vi "Pre Launch Init.vi"(11 "Rack Controller in":refnum<class "Rack Controller.lvclass">) -> (0 "error out":errorcluster, 3 "Rack Controller out":refnum<class "Rack Controller.lvclass">)   [LabVIEW 2019, in "Rack Controller.lvclass"]
doc: "(<B>Filename</B>: Actor Framework.lvlib:Actor.lvclass:Pre Launch Init.vi)\n\nDefines behavior that occurs after the Launch Nested Actor method is invoked but before the actor's Actor Core method begins running.\n\nBy default, this method does nothing. A descendant class may override it to define behavior."
uses:
  Rack Controller.lvclass
  <vilib>/ActorFramework/Message Enqueuer/Message Enqueuer.lvclass
  <vilib>/vision/Image Controls.llb/IMAQ Image.ctl
  <vilib>/ActorFramework/Actor/Actor.lvclass
  Common/Controls/Acknowledgement.ctl
  Common/Controls/Camera Optics Diagnostics.ctl
  Common/Controls/Camera Optics Diagnostics Result.ctl
  Common/Controls/Camera Info.ctl
  Inspection Statemachine/Controls/Result Cluster_SM.ctl
  Inspection Statemachine/Inspection Statemachine.lvclass
  Controls/Result Cluster_RC.ctl
  Common/Controls/AllPartInfo.ctl
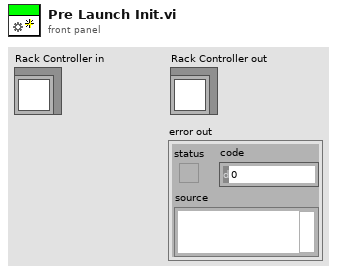
[diagram p1: front panel]
types:
  T1 = typedef "IMAQ Image.ctl" = refnum<image>
  T2 = typedef "AllPartInfo.ctl" = cluster{"PartName":string, "NumberOfRacks":u8, "MeasurementIDsArray":u16[], "MeasurementNamesArray":string[], "SpecValuesArray":cluster{"LCL":dbl, "UCL":dbl, "LSL":dbl, "USL":dbl, "NominalValue":dbl}[]}[]
  T3 = cluster{"PartName":string, "MeasurementIDsArray":u16[], "MeasurementNamesArray":string[], "SpecValuesArray":cluster{"LCL":dbl, "UCL":dbl, "LSL":dbl, "USL":dbl, "NominalValue":dbl}[]}
  T4 = cluster{"Unload Position Counts":cluster{"Fail":u32, "ReelEnd":u32, "ProductionEnd":u32}, "Number of Cameras":u8}
  T5 = cluster{"Result Cluster":cluster{"Rack ID":u8, "Measurement Values Array ":dbl[], "Images Array":T1[], "Result PF":bool, "Production Count Details":cluster{"Total Fail":u64, "Total Pass":u64, "Total Count":u64}, "Reel Count Details":cluster{"Reel Fail":u64, "Reel Pass":u64, "Reel Count":u64}, "Control PF Array":bool[], "Specification PF Array":bool[], "Specification Fail?":bool, "Reel Number":u64, "Status":string}, "Pause on Fail?":bool, "Total Count Finish?":bool, "Reel Count Finish?":bool}
  T6 = typedef "Inspection Statemachine.lvclass/Result Cluster_SM.ctl" = cluster{"RackID":u8, "MeasurementValuesArray ":dbl[], "ImagesArray":T1[], "ResultPF":bool, "ProductionCountDetails":cluster{"TotalFail":u64, "TotalPass":u64, "TotalCount":u64}, "ReelCountDetails":cluster{"ReelFail":u64, "ReelPass":u64, "ReelCount":u64}, "ControlPFArray":bool[], "SpecificationPFArray":bool[], "SpecificationFail":bool, "ReelNumber":u64, "Status":string}
  T7 = cluster{"Part Name":string, "Total Count":u64, "Reel Count":u64}
  T8 = typedef "Camera Info.ctl" = cluster{"Camera Names":string[], "Number of Active Cameras":u8}
  T9 = typedef "Camera Optics Diagnostics Result.ctl" = cluster{"LightCameraName":string, "DiagnosedImage":T1, "DustPercentage":dbl, "Result":bool}
  T10 = typedef "Camera Optics Diagnostics.ctl" = cluster{"Light Camera Name":string, " State":string}
  T11 = typedef "Rack Controller.lvclass/Result Cluster_RC.ctl" = cluster{"Measurement Values Array ":dbl[], "Images Array":T1[], "Result PF":bool, "Production Count Details":cluster{"Total Fail":u64, "Total Pass":u64, "Total Count":u64}, "Reel Count Details":cluster{"Reel Fail":u64, "Reel Pass":u64, "Reel Count":u64}, "Control PF Array":bool[], "Specification PF Array":bool[], "Specification Fail?":bool}
  T12 = typedef "Acknowledgement.ctl" = cluster{"Enqueuer":refnum<class "Message Enqueuer.lvclass">, "VIReference":refnum<vi>, "VIName":string}
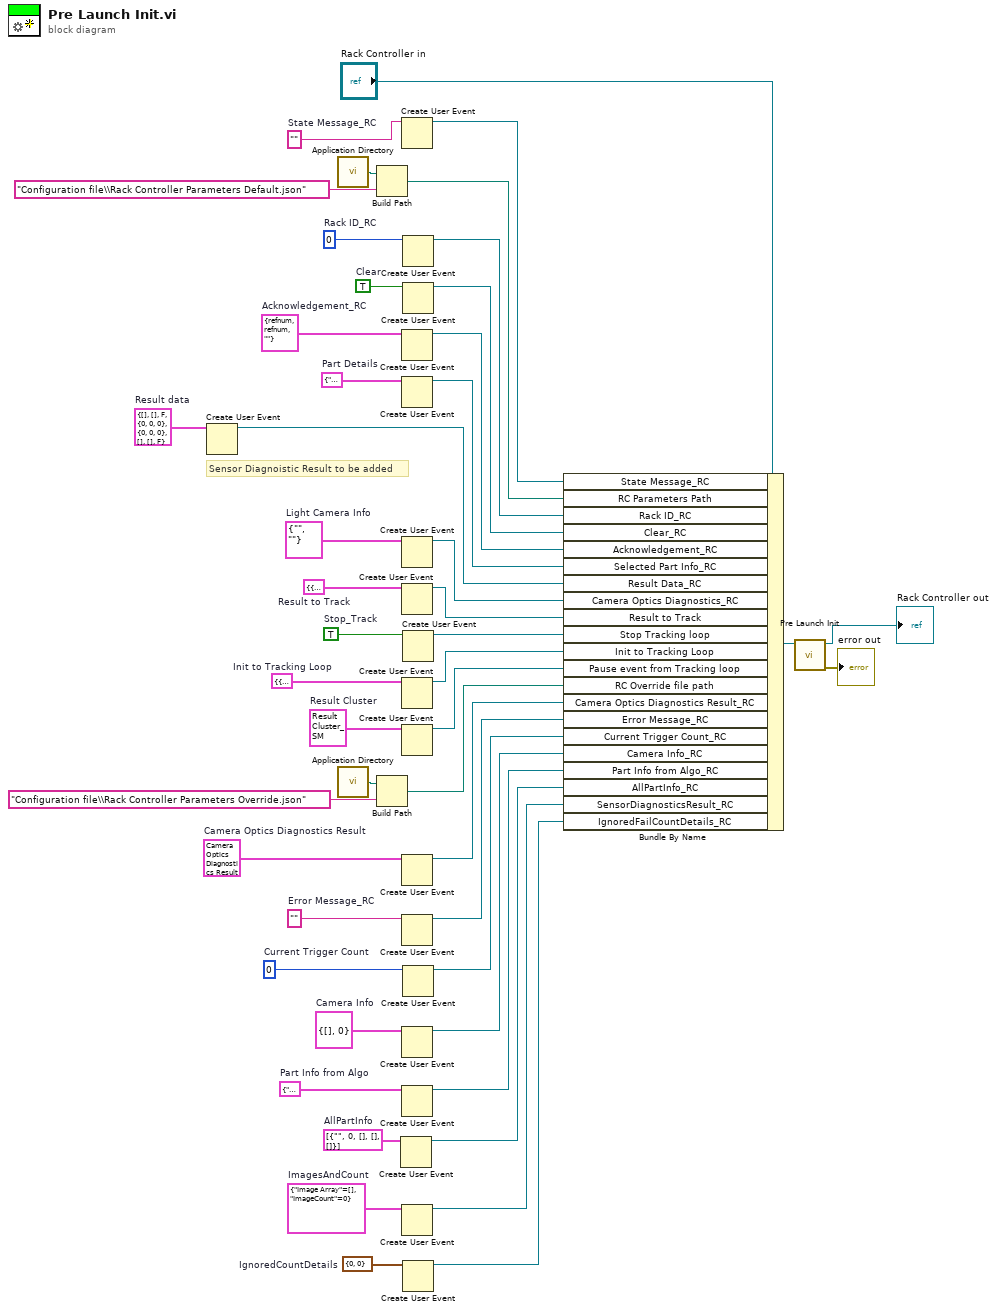
[diagram p0: block diagram]
diagram:
  w2 = cluster{"ReelCount":u64, "TotalCount":u64} {"ReelCount"=0, "TotalCount"=0}  # IgnoredCountDetails
  w4 = cluster{"Image Array":T1[], "ImageCount":u64} {"Image Array"=[], "ImageCount"=0}  # ImagesAndCount
  w6 = T2 [{"PartName"="", "NumberOfRacks"=0, "MeasurementIDsArray"=[], "MeasurementNamesArray"=[], "SpecValuesArray"=[]}]  # AllPartInfo
  w8 = T3 {"PartName"="", "MeasurementIDsArray"=[], "MeasurementNamesArray"=[], "SpecValuesArray"=[]}  # Part Info from Algo
  w13 = T4 {"Unload Position Counts"={"Fail"=0, "ReelEnd"=0, "ProductionEnd"=0}, "Number of Cameras"=0}  # Init to Tracking Loop
  w15 = T5 {"Result Cluster"={"Rack ID"=0, "Measurement Values Array "=[], "Images Array"=[], "Result PF"=FALSE, "Production Count Details"={"Total Fail"=0, "Total Pass"=0, "Total Count"=0}, "Reel Count Details"={"Reel Fail"=0, "Reel Pass"=0, "Reel Count"=0}, "Control PF Array"=[], "Specification PF Array"=[], "Specification Fail?"=FALSE, "Reel Number"=0, "Status"=""}, "Pause on Fail?"=TRUE, "Total Count Finish?"=FALSE, "Reel Count Finish?"=FALSE}  # Result to Track
  w11 = T6 {"RackID"=0, "MeasurementValuesArray "=[], "ImagesArray"=[], "ResultPF"=FALSE, "ProductionCountDetails"={"TotalFail"=0, "TotalPass"=0, "TotalCount"=0}, "ReelCountDetails"={"ReelFail"=0, "ReelPass"=0, "ReelCount"=0}, "ControlPFArray"=[], "SpecificationPFArray"=[], "SpecificationFail"=FALSE, "ReelNumber"=0, "Status"=""}  # Result Cluster
  w18 = T7 {"Part Name"="", "Total Count"=0, "Reel Count"=0}  # Part Details
  w21 = T8 {"Camera Names"=[], "Number of Active Cameras"=0}  # Camera Info
  w25 = T9 {"LightCameraName"="", "DiagnosedImage"=refnum, "DustPercentage"=0.0, "Result"=TRUE}  # Camera Optics Diagnostics Result
  w29 = u64 0  # Current Trigger Count
  w31 = ""  # Error Message_RC
  w36 = TRUE  # Stop_Track
  w37 = T10 {"Light Camera Name"="", " State"=""}  # Light Camera Info
  w10 = T11 {"Measurement Values Array "=[], "Images Array"=[], "Result PF"=FALSE, "Production Count Details"={"Total Fail"=0, "Total Pass"=0, "Total Count"=0}, "Reel Count Details"={"Reel Fail"=0, "Reel Pass"=0, "Reel Count"=0}, "Control PF Array"=[], "Specification PF Array"=[], "Specification Fail?"=FALSE}  # Result data
  w41 = T12 {"Enqueuer"=refnum, "VIReference"=refnum, "VIName"=""}  # Acknowledgement_RC
  w42 = TRUE  # Clear
  w43 = 0  # Rack ID_RC
  w44 = ""  # State Message_RC
  # "Sensor Diagnoistic Result to be added"
  n1 = Create User Event(user event datatype=w10) -> (user event=w28:refnum<user-event>)  [unwired: 1 in, 1 out]
  n2 = call <vilib>:"Application Directory.vi"() -> ("Application Directory"=w40:path)
  n3 = call <vilib>:"Application Directory.vi"() -> ("Application Directory"=w34:path)
  n4 = Build Path(base path=w40, name or relative path="Configuration file\\Rack Controller Parameters Default.json") -> (appended path=w38:path)
  n5 = Build Path(base path=w34, name or relative path="Configuration file\\Rack Controller Parameters Override.json") -> (appended path=w32:path)
  n6 = Create User Event(user event datatype=w6) -> (user event=w5:refnum<user-event>)  [unwired: 1 in, 1 out]
  n7 = Create User Event(user event datatype=w44) -> (user event=w19:refnum<user-event>)  [unwired: 1 in, 1 out]
  n8 = Create User Event(user event datatype=w41) -> (user event=w27:refnum<user-event>)  [unwired: 1 in, 1 out]
  n9 = Create User Event(user event datatype=w18) -> (user event=w17:refnum<user-event>)  [unwired: 1 in, 1 out]
  n10 = Create User Event(user event datatype=w37) -> (user event=w26:refnum<user-event>)  [unwired: 1 in, 1 out]
  n11 = Create User Event(user event datatype=w15) -> (user event=w14:refnum<user-event>)  [unwired: 1 in, 1 out]
  n12 = Create User Event(user event datatype=w13) -> (user event=w12:refnum<user-event>)  [unwired: 1 in, 1 out]
  n13 = Create User Event(user event datatype=w11) -> (user event=w16:refnum<user-event>)  [unwired: 1 in, 1 out]
  n14 = Create User Event(user event datatype=w25) -> (user event=w24:refnum<user-event>)  [unwired: 1 in, 1 out]
  n15 = Create User Event(user event datatype=w31) -> (user event=w30:refnum<user-event>)  [unwired: 1 in, 1 out]
  n16 = Create User Event(user event datatype=w21) -> (user event=w20:refnum<user-event>)  [unwired: 1 in, 1 out]
  n17 = Create User Event(user event datatype=w8) -> (user event=w7:refnum<user-event>)  [unwired: 1 in, 1 out]
  n18 = Create User Event(user event datatype=w4) -> (user event=w3:refnum<user-event>)  [unwired: 1 in, 1 out]
  n19 = Create User Event(user event datatype=w43) -> (user event=w23:refnum<user-event>)  [unwired: 1 in, 1 out]
  n20 = Create User Event(user event datatype=w42) -> (user event=w22:refnum<user-event>)  [unwired: 1 in, 1 out]
  n21 = Create User Event(user event datatype=w36) -> (user event=w35:refnum<user-event>)  [unwired: 1 in, 1 out]
  n22 = Create User Event(user event datatype=w29) -> (user event=w9:refnum<user-event>)  [unwired: 1 in, 1 out]
  n23 = Create User Event(user event datatype=w2) -> (user event=w1:refnum<user-event>)  [unwired: 1 in, 1 out]
  n24 = Bundle By Name(cluster="Rack Controller in", "State Message_RC"=w19, "RC Parameters Path"=w38, "Rack ID_RC"=w23, "Clear_RC"=w22, "Acknowledgement_RC"=w27, "Selected Part Info_RC"=w17, "Result Data_RC"=w28, "Camera Optics Diagnostics_RC"=w26, "Result to Track"=w14, "Stop Tracking loop"=w35, "Init to Tracking Loop"=w12, "Pause event from Tracking loop"=w16, "RC Override file path"=w32, "Camera Optics Diagnostics Result_RC"=w24, "Error Message_RC"=w30, "Current Trigger Count_RC"=w9, "Camera Info_RC"=w20, "Part Info from Algo_RC"=w7, "AllPartInfo_RC"=w5, "SensorDiagnosticsResult_RC"=w3, "IgnoredFailCountDetails_RC"=w1) -> (w45:refnum<class "Rack Controller.lvclass">)
  n25 = call-parent "Pre Launch Init.vi"("Actor in"=w45) -> ("error out"=→"error out":errorcluster, "Actor out"=→"Rack Controller out":refnum<class "Rack Controller.lvclass">)  [unwired: 9 in]
